vi "ReadDataVariant.vi"(8 "error in (no error)":errorcluster, 11 "Singleton.lvclass In":refnum<class "Singleton.lvclass">) -> (0 "error out":errorcluster, 2 "DataVariant":variant, 3 "SingletonDVR Out":refnum<data-value>)   [LabVIEW 2013, in "Singleton.lvclass"]
uses:
  Singleton.lvclass
  Singleton.lvclass/Singleton.ctl
panel:
  # "ReadDataVariant"
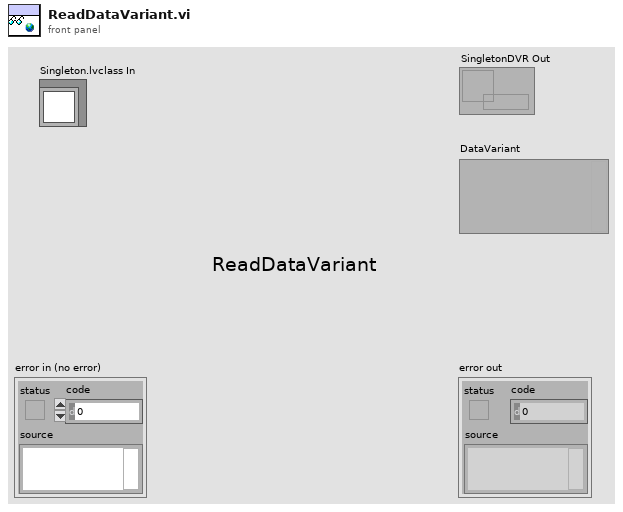
[diagram p1: front panel]
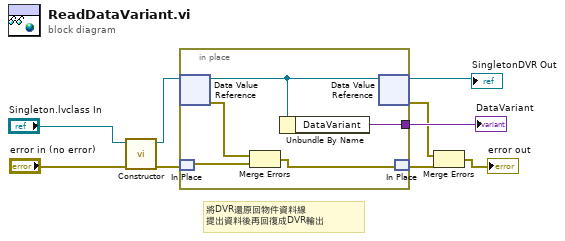
[diagram p0: block diagram]
diagram:
  # "將DVR還原回物件資料線\n提出資料後再回復成DVR輸出"
  n1 = call "Constructor.vi"("error in (no error)"="error in (no error)", "Singleton.lvclass In"="Singleton.lvclass In") -> ("error out"=w2:errorcluster, "SingletonDVR Out"=w1:refnum<data-value>)  [unwired: 8 in]
  n2 = in-place {
    in-place-border: [w10] -> w8
    n3 = in-place-dvr #1(w1) -> (w11:refnum<class "Singleton.lvclass">, w13:errorcluster)
    n4 = in-place-match #2(w2) -> (w14:errorcluster)
    n5 = Merge Errors(w13, w14) -> (w12:errorcluster)
    n6 = Unbundle By Name(w11) -> ("DataVariant"=w10:variant)
    n7 = in-place-dvr #1(w11) -> (→"SingletonDVR Out":refnum<data-value>, w6:errorcluster)
    n8 = in-place-match #2(w12) -> (w7:errorcluster)
  }
  "DataVariant" <- w8
  n9 = Merge Errors(w6, w7) -> (→"error out":errorcluster)
